vi "FuzzyEx Dynamic Fuzzy Controller for a greenhouse.vi"() -> ()   [LabVIEW 2023]
doc: "This example illustrates how to use a fuzzy controller to control a greenhouse system."
uses:
  <vilib>/addons/Fuzzy Logic/TypeDefs/FL System.ctl
  <vilib>/addons/Fuzzy Logic/TypeDefs/FL Variable.ctl
  <vilib>/addons/Fuzzy Logic/TypeDefs/FL Membership Function.ctl
  <vilib>/addons/Fuzzy Logic/TypeDefs/FL Membership Function Shape.ctl
  <vilib>/addons/Fuzzy Logic/TypeDefs/FL Rule.ctl
  <vilib>/addons/Fuzzy Logic/TypeDefs/FL Antecedent.ctl
  <vilib>/addons/Fuzzy Logic/TypeDefs/FL Modifier.ctl
  <vilib>/addons/Fuzzy Logic/TypeDefs/FL Antecedent Connective.ctl
  <vilib>/addons/Fuzzy Logic/TypeDefs/FL Consequent.ctl
  <vilib>/addons/Fuzzy Logic/TypeDefs/FL Consequent Implication.ctl
  <vilib>/addons/Fuzzy Logic/TypeDefs/FL Defuzzification.ctl
  <vilib>/addons/Fuzzy Logic/TypeDefs/FL Interpolating polynomials.ctl
  <vilib>/addons/Fuzzy Logic/TypeDefs/FL Input_Output.ctl
  <vilib>/addons/Fuzzy Logic/FL Fuzzy Controller (MIMO).vi
  <vilib>/addons/Fuzzy Logic/Membership/FL Get Membership Function (Fuzzy System).vi
  <vilib>/addons/Fuzzy Logic/Membership/FL Set Membership Function (Fuzzy System).vi
  <vilib>/addons/Fuzzy Logic/NI_Fuzzy_Logic_API.lvlib
panel:
  out "fuzzy system out":T1={"input variables"=[{"name"="Temperature", "range"=[0.0, 50.0, 0.0, 50.0], "MFs"=[{"name"="Cold", "shape"=1, "points"=[0.0, 0.0, 13.0, 21.0], "color"=42751, "user-defined shape index"=0}, {"name"="Normal", "shape"=3, "points"=[15.0, 20.0, 25.0, 30.0], "color"=16757760, "user-defined shape index"=0}, {"name"="Warm", "shape"=1, "points"=[24.0, 32.0, 50.0, 50.0], "color"=16714752, "user-defined shape index"=0}]}, {"name"="Humidity", "range"=[0.0, 100.0, 0.0, 100.0], "MFs"=[{"name"="Dry", "shape"=4, "points"=[0.0, 0.0, 10.0, 70.0], "color"=11796480, "user-defined shape index"=0}, {"name"="Normal", "shape"=4, "points"=[15.0, 68.0, 75.0, 90.0], "color"=16759338, "user-defined shape index"=0}, {"name"="Wet", "shape"=3, "points"=[70.0, 90.0, 100.0, 100.0], "color"=11861920, "user-defined shape index"=0}]}], "output variables"=[{"name"="Electric Roof", "range"=[0.0, 10.0, 0.0, 10.0], "MFs"=[{"name"="Closed", "shape"=0, "points"=[0.0, 0.0, 5.0], "color"=16711680, "user-defined shape index"=0}, {"name"="Semi-open", "shape"=0, "points"=[0.0, 5.0, 10.0], "color"=16774656, "user-defined shape index"=0}, {"name"="Open", "shape"=0, "points"=[5.0, 10.0, 10.0], "color"=2410496, "user-defined shape index"=0}]}, {"name"="Water Spills", "range"=[0.0, 10.0, 0.0, 10.0], "MFs"=[{"name"="Less", "shape"=0, "points"=[0.0, 0.0, 5.0], "color"=15263, "user-defined shape index"=0}, {"name"="Moderate", "shape"=0, "points"=[0.0, 5.0, 10.0], "color"=34559, "user-defined shape index"=0}, {"name"="More", "shape"=0, "points"=[5.0, 10.0, 10.0], "color"=2811647, "user-defined shape index"=0}]}], "rules"=[{"antecedents"=[{"Var Index"=0, "MF Index"=0, "Cond"=0}, {"Var Index"=1, "MF Index"=0, "Cond"=0}], "antecedent connective"=0, "consequents"=[{"Var Index"=0, "MF Index"=0, "Cond"=0}, {"Var Index"=1, "MF Index"=1, "Cond"=0}], "consequent implication"=1, "degree of support"=1.0}, {"antecedents"=[{"Var Index"=0, "MF Index"=0, "Cond"=0}, {"Var Index"=1, "MF Index"=1, "Cond"=0}], "antecedent connective"=0, "consequents"=[{"Var Index"=0, "MF Index"=0, "Cond"=0}, {"Var Index"=1, "MF Index"=0, "Cond"=0}], "consequent implication"=1, "degree of support"=1.0}, {"antecedents"=[{"Var Index"=0, "MF Index"=0, "Cond"=0}, {"Var Index"=1, "MF Index"=2, "Cond"=0}], "antecedent connective"=0, "consequents"=[{"Var Index"=0, "MF Index"=0, "Cond"=0}, {"Var Index"=1, "MF Index"=0, "Cond"=0}], "consequent implication"=1, "degree of support"=1.0}, {"antecedents"=[{"Var Index"=0, "MF Index"=1, "Cond"=0}, {"Var Index"=1, "MF Index"=0, "Cond"=0}], "antecedent connective"=0, "consequents"=[{"Var Index"=0, "MF Index"=1, "Cond"=0}, {"Var Index"=1, "MF Index"=2, "Cond"=0}], "consequent implication"=1, "degree of support"=1.0}, {"antecedents"=[{"Var Index"=0, "MF Index"=1, "Cond"=0}, {"Var Index"=1, "MF Index"=1, "Cond"=0}], "antecedent connective"=0, "consequents"=[{"Var Index"=0, "MF Index"=1, "Cond"=0}, {"Var Index"=1, "MF Index"=1, "Cond"=0}], "consequent implication"=1, "degree of support"=1.0}, {"antecedents"=[{"Var Index"=0, "MF Index"=1, "Cond"=0}, {"Var Index"=1, "MF Index"=2, "Cond"=0}], "antecedent connective"=0, "consequents"=[{"Var Index"=0, "MF Index"=1, "Cond"=0}, {"Var Index"=1, "MF Index"=0, "Cond"=0}], "consequent implication"=1, "degree of support"=1.0}, {"antecedents"=[{"Var Index"=0, "MF Index"=2, "Cond"=0}, {"Var Index"=1, "MF Index"=0, "Cond"=0}], "antecedent connective"=0, "consequents"=[{"Var Index"=0, "MF Index"=2, "Cond"=0}, {"Var Index"=1, "MF Index"=2, "Cond"=0}], "consequent implication"=1, "degree of support"=1.0}, {"antecedents"=[{"Var Index"=0, "MF Index"=2, "Cond"=0}, {"Var Index"=1, "MF Index"=1, "Cond"=0}], "antecedent connective"=0, "consequents"=[{"Var Index"=0, "MF Index"=2, "Cond"=0}, {"Var Index"=1, "MF Index"=1, "Cond"=0}], "consequent implication"=1, "degree of support"=1.0}, {"antecedents"=[{"Var Index"=0, "MF Index"=2, "Cond"=0}, {"Var Index"=1, "MF Index"=2, "Cond"=0}], "antecedent connective"=0, "consequents"=[{"Var Index"=0, "MF Index"=2, "Cond"=0}, {"Var Index"=1, "MF Index"=1, "Cond"=0}], "consequent implication"=1, "degree of support"=1.0}], "defuzzification method"=3, "description"="", "user MF interpolating polynomials"=[]} {"user MF interpolating polynomials"."coa_x(y) coeff" format="%.4g"; "user MF interpolating polynomials"."Area(y) coeff" format="%.4g"; "user MF interpolating polynomials"."X(y) coeff" format="%.4g"; "user MF interpolating polynomials"."Y(x) coeff" format="%.4g"; "user MF interpolating polynomials"."Y" format="%.4g"; "user MF interpolating polynomials"."X" format="%.4g"; "defuzzification method" items=["Center of Area", "Modified Center of Area", "Center of Sums", "Center of Maximum", "Mean of Maximum"]; "rules"."consequents"."Var Index" min=0; "rules"."consequents"."Cond" items=["=", "!="]; "rules"."consequents"."MF Index" min=0; "rules"."antecedents"."Var Index" min=0; "rules"."antecedents"."Cond" items=["=", "!="]; "rules"."antecedents"."MF Index" min=0; "rules"."consequent implication" items=["Minimum", "Product"]; "rules"."antecedent connective" items=["AND (Minimum)", "AND (Product)", "OR (Maximum)", "OR (Probabilistic)"]; "output variables"."MFs"."shape" items=["Triangle", "Trapezoid", "Singleton", "Sigmoid", "Gaussian", "User-Defined"]; "input variables"."MFs"."shape" items=["Triangle", "Trapezoid", "Singleton", "Sigmoid", "Gaussian", "User-Defined"]}
  in  "Tab Control":enum32{"Introduction", "Dynamic Controller"}(tab)
  in  "Temperature (deg C)":dbl(slide)=25.0 scale=0.0..50.0
  in  "Humidity (%)":dbl(slide)=70.0 scale=0.0..100.0
  out "Roof Opening (%)":dbl(slide)=5.555555555555555 scale=0.0..10.0
  out "Water Spills (%)":dbl(slide)=4.976391598507772 scale=0.0..10.0
  in  "Season":dbl(knob) scale=5.0..-10.0
  out "Membership functions for temperature":cluster{cluster{"Xi":dbl, "Yi":dbl}[]}[](graph)
  in  "Stop":bool
  # "IF"
  # "THEN"
  # "Overview: The Green Engineering concepts are used in this example to illustrate how to build a dynamic Fuzzy Logic Controller. Greenhouses are used to cultivate plants by continuously maintaining good conditions for growth throughout the year. The challenge of using devices to control the environment is to have a consistent controller that can adapt to any weather condition.\nFuzzy Logic can be used to describe a controller for a process like this. On the other hand, it becomes difficult to create controller Rules for every climatic condition, and a good strategy is to create dynamic controllers.\nA dynamic controller can change its parameter on the fly, without stopping controller action, and in this case is presented a controller that can shift its membership functions to adapt itself to the temperatures in every weather season.\nIn the summer, the average temperatures are higher. In the winter, the average temperatures are lower, and so on.\nInstructions:\n1. Run the VI.\n2. On the Dynamic Controller tab, experiment with different input parameters and see how the outputs change if you dynamically change the season.\n3. Click Stop to stop the VI."
  # "Dynamic Changes"
  # "Fuzzy\nController"
  # "sensors"
  # "actuators"
  # "Spring"
  # "Fall"
  # "Summer"
  # "Winter"
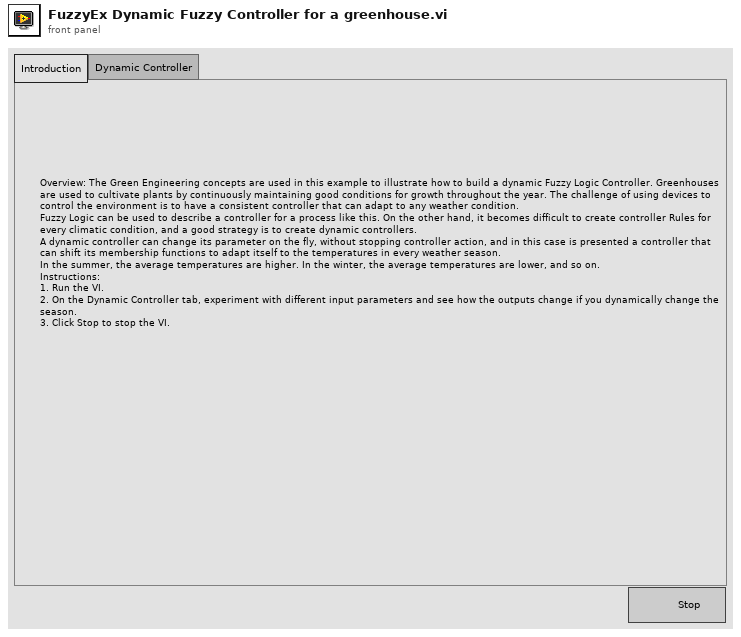
[diagram p1: front panel]
types:
  T1 = typedef "NI_Fuzzy_Logic_API.lvlib/FL System.ctl" = cluster{"input variables":T2[], "output variables":T2[], "rules":T5[], "defuzzification method":T11, "description":string, "user MF interpolating polynomials":T12[]}
  T2 = typedef "NI_Fuzzy_Logic_API.lvlib/FL Variable.ctl" = cluster{"name":string, "range":dbl[], "MFs":T3[]}
  T3 = typedef "NI_Fuzzy_Logic_API.lvlib/FL Membership Function.ctl" = cluster{"name":string, "shape":T4, "points":dbl[], "color":u32, "user-defined shape index":i32}
  T4 = typedef "NI_Fuzzy_Logic_API.lvlib/FL Membership Function Shape.ctl" = u16
  T5 = typedef "NI_Fuzzy_Logic_API.lvlib/FL Rule.ctl" = cluster{"antecedents":T6[], "antecedent connective":T8, "consequents":T9[], "consequent implication":T10, "degree of support":dbl}
  T6 = typedef "NI_Fuzzy_Logic_API.lvlib/FL Antecedent.ctl" = cluster{"Var Index":i32, "MF Index":i32, "Cond":T7}
  T7 = typedef "NI_Fuzzy_Logic_API.lvlib/FL Modifier.ctl" = u16
  T8 = typedef "NI_Fuzzy_Logic_API.lvlib/FL Antecedent Connective.ctl" = u16
  T9 = typedef "NI_Fuzzy_Logic_API.lvlib/FL Consequent.ctl" = cluster{"Var Index":i32, "MF Index":i32, "Cond":T7}
  T10 = typedef "NI_Fuzzy_Logic_API.lvlib/FL Consequent Implication.ctl" = u16
  T11 = typedef "NI_Fuzzy_Logic_API.lvlib/FL Defuzzification.ctl" = u16
  T12 = typedef "NI_Fuzzy_Logic_API.lvlib/FL Interpolating polynomials.ctl" = cluster{"X":dbl[], "Y":dbl[], "Y(x) coeff":dbl[][], "X(y) coeff":dbl[][], "Area(y) coeff":dbl[][], "coa_x(y) coeff":dbl[][]}
  T13 = typedef "NI_Fuzzy_Logic_API.lvlib/FL Input_Output.ctl" = u16
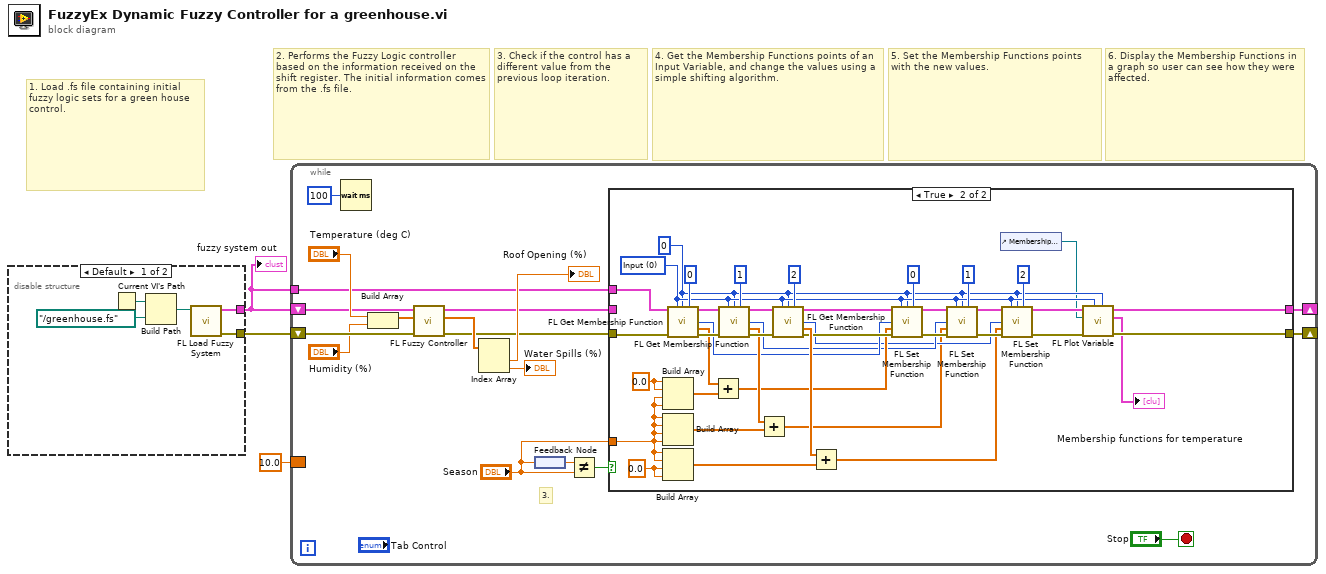
[diagram p0: block diagram]
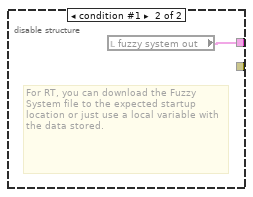
[diagram p2: hidden frame]
diagram:
  # "5. Set the Membership Functions points with the new values."
  # "4. Get the Membership Functions points of an Input Variable, and change the values using a simple shifting algorithm."
  # "3. Check if the control has a different value from the previous loop iteration."
  # "2. Performs the Fuzzy Logic controller based on the information received on the shift register. The initial information comes from the .fs file."
  # "1. Load .fs file containing initial fuzzy logic sets for a green house control."
  # "6. Display the Membership Functions in a graph so user can see how they were affected."
  n1 = disable-structure shown="Default" {
    disable-tunnel: [w8 _] -> w3
    disable-tunnel: [w7 w9] -> w2
    frame condition #0 (active) {
      n2 = Current VI's Path() -> (path=w6:path)
      n3 = Build Path(base path=w6, name or relative path=path "../greenhouse.fs") -> (appended path=w4:path)
      n4 = call <vilib>:"FL Load Fuzzy System.vi"("file path"=w4) -> ("error out"=w8:errorcluster, "fuzzy system out"=w7:T1)  [unwired: 1 in, 8 out]
    }
    frame condition #1 {
      # "For RT, you can download the Fuzzy System file to the expected startup location or just use a local variable with the data stored."
      n5 = local read "fuzzy system out"() -> (w9:T1)
    }
  }
  "fuzzy system out" <- w2
  n6 = while {
    shift-right: [w13] -> _
    shift-left: w2 -> [w11]
    shift-right: [w14] -> _
    shift-left: w3 -> [w26]
    tunnel: w2 -> [w10]
    border: 10.0 ("Season") -> [_]
    stop <- "Stop" stop-if-true
    # "3."
    n7 = Wait (ms)(milliseconds to wait=u32 100) -> ()  [unwired: 1 out]
    n8 = Build Array("Temperature (deg C)", "Humidity (%)") -> (w23:dbl[])
    n9 = call-poly <vilib>:"FL Fuzzy Controller.vi"("error in (no error)"=w26, "input values"=w23, "fuzzy system in"=w11) -> ("error out"=w15:errorcluster, "output values"=w22:dbl[], "fuzzy system out"=w16:T1)  [unwired: 6 out]
    n10 = Index Array(array=w22) -> (element #1=→"Roof Opening (%)":dbl, element #2=→"Water Spills (%)":dbl)  [unwired: 2 in]
    n11 = feedback-in #1("Season") -> ()
    n12 = feedback #1() -> (w18:dbl)
    n13 = Not Equal?(x=w18, y="Season") -> (x != y?=w17:bool)
    n14 = case shown="True" w17 {
      tunnel: w16 -> [w29 _]
      tunnel: w15 -> [w28 w70]
      tunnel: [w28 w34] -> w14
      tunnel: [w29 w36] -> w13
      tunnel: "Season" -> [_ w64]
      tunnel: w10 -> [_ w69]
      frame False {
        # "Does not change controller parameters if not needed"
      }
      frame True {
        w43 = 0.0 ("element")
        w45 = 0.0 ("element")
        w32 = 0 ("Var index")
        w33 = T13 0 items=["Input", "Output"] ("Input/Output")
        n15 = Build Array(w45, w45, w64, w64) -> (w62:dbl[])
        n16 = Build Array(w64, w64, w64, w64) -> (w61:dbl[])
        n17 = Build Array(w64, w64, w43, w43) -> (w59:dbl[])
        n18 = call-poly <vilib>:"FL Get Membership Function.vi"("fuzzy system in"=w69, "input/output"=w33, "variable index"=w32, "membership function index"=0 ("MF index"), "error in (no error)"=w70) -> ("fuzzy system out"=w68:T1, "shape"=w48:T4, "points"=w63:dbl[], "error out"=w67:errorcluster)  [unwired: 7 out]
        n19 = Add(x=w63, y=w62) -> (x+y=w50:dbl[])
        n20 = call-poly <vilib>:"FL Get Membership Function.vi"("fuzzy system in"=w68, "input/output"=w33, "variable index"=w32, "membership function index"=1 ("MF index"), "error in (no error)"=w67) -> ("fuzzy system out"=w66:T1, "shape"=w47:T4, "points"=w60:dbl[], "error out"=w65:errorcluster)  [unwired: 7 out]
        n21 = Add(x=w60, y=w61) -> (x+y=w44:dbl[])
        n22 = call-poly <vilib>:"FL Get Membership Function.vi"("fuzzy system in"=w66, "input/output"=w33, "variable index"=w32, "membership function index"=2 ("MF index"), "error in (no error)"=w65) -> ("fuzzy system out"=w57:T1, "shape"=w46:T4, "points"=w58:dbl[], "error out"=w56:errorcluster)  [unwired: 7 out]
        n23 = Add(x=w58, y=w59) -> (x+y=w49:dbl[])
        n24 = call-poly <vilib>:"FL Set Membership Function.vi"("fuzzy system in"=w57, "input/output"=w33, "variable index"=w32, "membership function index"=0 ("MF index"), "shape"=w48, "points"=w50, "error in (no error)"=w56) -> ("fuzzy system out"=w53:T1, "error out"=w52:errorcluster)  [unwired: 3 in, 4 out]
        n25 = call-poly <vilib>:"FL Set Membership Function.vi"("fuzzy system in"=w53, "input/output"=w33, "variable index"=w32, "membership function index"=1 ("MF index"), "shape"=w47, "points"=w44, "error in (no error)"=w52) -> ("fuzzy system out"=w55:T1, "error out"=w54:errorcluster)  [unwired: 3 in, 4 out]
        n26 = control-ref of="Membership functions for temperature"() -> (w31:refnum<vi>)
        n27 = call-poly <vilib>:"FL Set Membership Function.vi"("fuzzy system in"=w55, "input/output"=w33, "variable index"=w32, "membership function index"=2 ("MF index"), "shape"=w46, "points"=w49, "error in (no error)"=w54) -> ("fuzzy system out"=w37:T1, "error out"=w35:errorcluster)  [unwired: 3 in, 4 out]
        n28 = call <vilib>:"FL Plot Variable.vi"("variable index"=w32, "input/output"=w33, "error in (no error)"=w35, "graph refnum"=w31, "fuzzy system in"=w37) -> ("error out"=w34:errorcluster, "membership functions plot"=→"Membership functions for temperature":cluster{cluster{"Xi":dbl, "Yi":dbl}[]}[], "fuzzy system out"=w36:T1)  [unwired: 4 out]
      }
    }
  }
